vi "histogram_lifetimes.vi"(8 "error in (no error)":errorcluster, 11 "swabian_local_data 2":T1={"events"={"update_status"=refnum, "update_chart"=refnum, "update_xy"=refnum, "send_channel_data"=refnum}, "stop_q"=refnum, "tagger_reference"=refnum, "connect_button"=refnum, "counter_reference"=refnum, "tagger_stream_reference"=refnum, "log_reference"=refnum, "current_log_offset"=0, "tt20_buffer_q"=refnum, "stream_to_file_button"=refnum, "num_records"=0, "connected?"=FALSE, "plots"=refnum, "histogram_bin_edges"=[], "histogrammer"=refnum, "plot_lifetimes"=refnum, "xy_graph"=refnum, "Reference\nChannel"=enum."ch0", "trigger_channels"=[], "filter_channels"=[], "active_channels"=[], "acq_mode"=0, "Reference\nChannel"=enum."ch0", "acq_time"=0, "sync_period_ps"=0, "raw_stream_path"=path "", "Leftovers"={"missing_sync_data"=[], "missing_events"=0}, "first_batch"=0, "first_sync_stamp"=0, "lifetime_settings"={"Plot Lifetimes"=FALSE, "start_time"=0.0, "stop_time"=0.0, "n_bins"=0, "Oscilloscope"=TRUE}, "Histogram_bins"=[], "last_processed_data"=[], "histogram_data"=[]}) -> (0 "error out":errorcluster, 3 "swabian_local_data 3":T1={"events"={"update_status"=refnum, "update_chart"=refnum, "update_xy"=refnum, "send_channel_data"=refnum}, "stop_q"=refnum, "tagger_reference"=refnum, "connect_button"=refnum, "counter_reference"=refnum, "tagger_stream_reference"=refnum, "log_reference"=refnum, "current_log_offset"=0, "tt20_buffer_q"=refnum, "stream_to_file_button"=refnum, "num_records"=0, "connected?"=FALSE, "plots"=refnum, "histogram_bin_edges"=[], "histogrammer"=refnum, "plot_lifetimes"=refnum, "xy_graph"=refnum, "Reference\nChannel"=enum."ch0", "trigger_channels"=[], "filter_channels"=[], "active_channels"=[], "acq_mode"=0, "Reference\nChannel"=enum."ch0", "acq_time"=0, "sync_period_ps"=0, "raw_stream_path"=path "", "Leftovers"={"missing_sync_data"=[], "missing_events"=0}, "first_batch"=0, "first_sync_stamp"=0, "lifetime_settings"={"Plot Lifetimes"=FALSE, "start_time"=0.0, "stop_time"=0.0, "n_bins"=0, "Oscilloscope"=TRUE}, "Histogram_bins"=[], "last_processed_data"=[], "histogram_data"=[]})   [LabVIEW 2018]
uses:
  swabian_local_data_tdef.ctl
  swabian_events_tdef.ctl
  update_chart_tdef.ctl
  channel_data_tdef.ctl
  C:/Users/SWIR TCSPC/Documents/swabian_LV/lib/TTCSharp32.dll
  lib/TTCSharp32.dll
  swabian_buffer_tdef.ctl
  reference_checkbox_tdef.ctl
  lifetime_settings.ctl
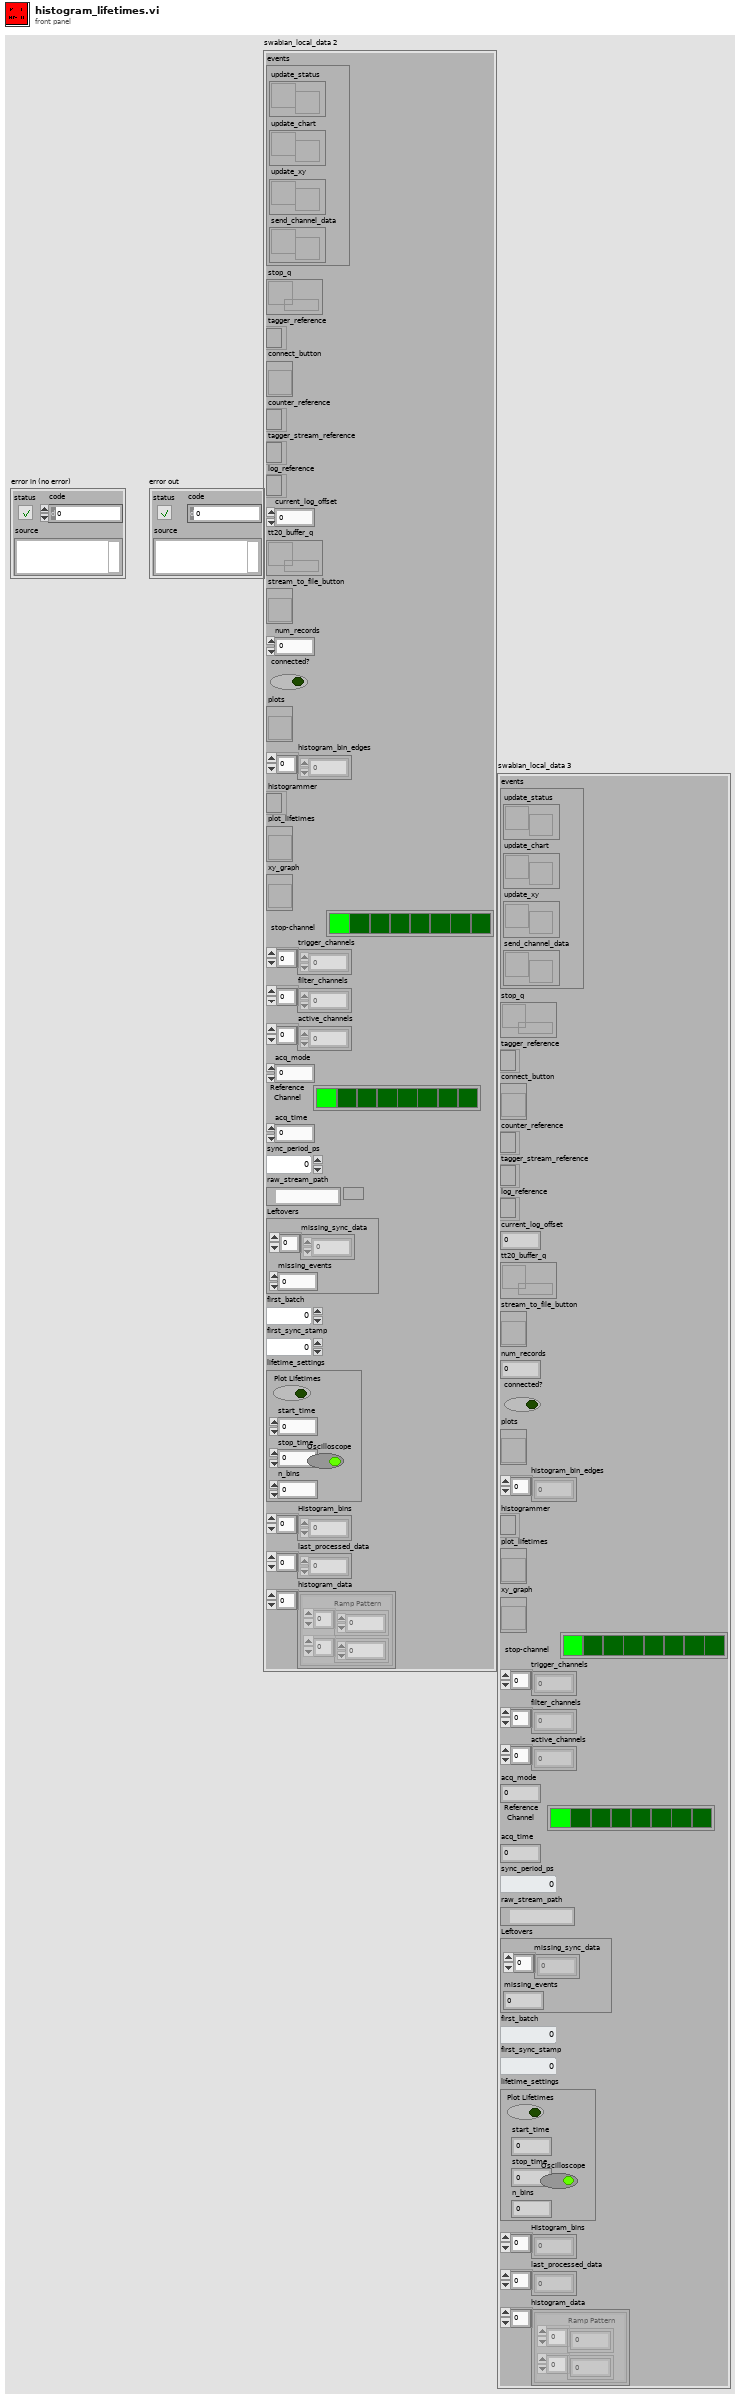
[diagram p1: front panel]
types:
  T1 = typedef "swabian_local_data_tdef.ctl" = cluster{"events":T2, "stop_q":refnum<queue>, "tagger_reference":refnum<k24>, "connect_button":refnum<vi>, "counter_reference":refnum<k24>, "tagger_stream_reference":refnum<k24>, "log_reference":refnum<file>, "current_log_offset":i64, "tt20_buffer_q":refnum<queue>, "stream_to_file_button":refnum<vi>, "num_records":u64, "connected?":bool, "plots":refnum<vi>, "histogram_bin_edges":i64[], "histogrammer":refnum<k24>, "plot_lifetimes":refnum<vi>, "xy_graph":refnum<vi>, "Reference\nChannel":T3, "trigger_channels":i32[], "filter_channels":i32[], "active_channels":i32[], "acq_mode":i32, "Reference\nChannel":T3, "acq_time":i64, "sync_period_ps":i64, "raw_stream_path":path, "Leftovers":cluster{"missing_sync_data":i64[], "missing_events":i32}, "first_batch":i32, "first_sync_stamp":i64, "lifetime_settings":T4, "Histogram_bins":dbl[], "last_processed_data":i64[], "histogram_data":cluster{"Ramp Pattern":dbl[], dbl[]}[]}
  T2 = typedef "swabian_events_tdef.ctl" = cluster{"update_status":refnum<user-event>, "update_chart":refnum<user-event>, "update_xy":refnum<user-event>, "send_channel_data":refnum<user-event>}
  T3 = typedef "reference_checkbox_tdef.ctl" = enum32{"No Selection", "ch0", "ch1", "ch2", "ch3", "ch4", "ch5", "ch6", "ch7"}
  T4 = typedef "lifetime_settings.ctl" = cluster{"Plot Lifetimes":bool, "start_time":dbl, "stop_time":dbl, "n_bins":i32, "Oscilloscope":bool}
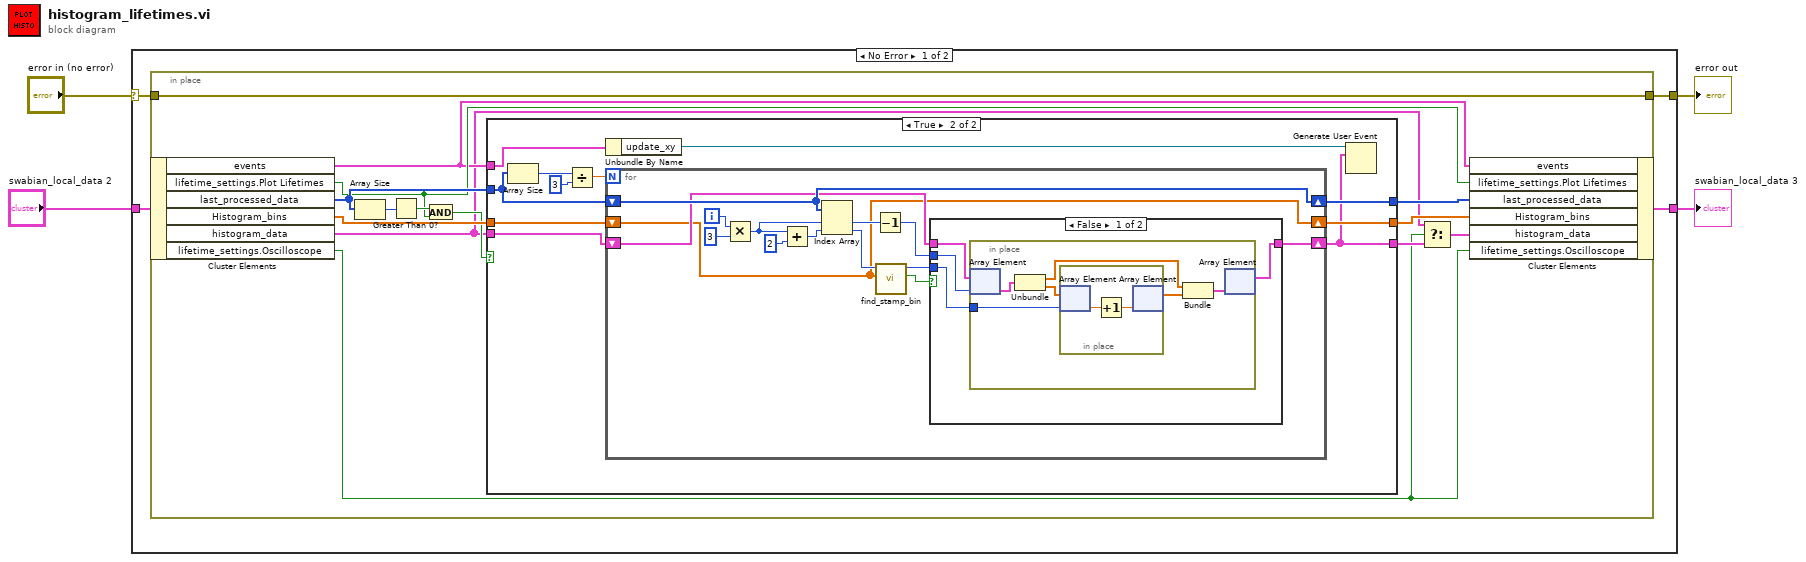
[diagram p0: block diagram]
diagram:
  n1 = case shown="No Error" "error in (no error)" {
    selector: "error in (no error)" -> [w7 w65]
    tunnel: "swabian_local_data 2" -> [w8 w64]
    tunnel: [w6 w65] -> w2
    tunnel: [w5 w64] -> w1
    frame No Error {
      n2 = in-place {
        in-place-border: w7 -> [w22]
        in-place-border: [w22] -> w6
        n3 = in-place-cluster #1(w8) -> ("events"=w13:T2, "lifetime_settings.Plot Lifetimes"=w15:bool, "last_processed_data"=w18:i64[], "Histogram_bins"=w21:dbl[], "histogram_data"=w10:cluster{"Ramp Pattern":dbl[], dbl[]}[], "lifetime_settings.Oscilloscope"=w9:bool)
        n4 = Array Size(array=w18) -> (size(s)=w17:i32)
        n5 = Greater Than 0?(x=w17) -> (x > 0?=w16:bool)
        n6 = And(x=w16, y=w15) -> (x .and. y?=w14:bool)
        n7 = case shown="True" w14 {
          tunnel: w13 -> [_ w36]
          tunnel: w18 -> [w25 w31]
          tunnel: w21 -> [w24 w30]
          tunnel: [w24 w29] -> w20
          tunnel: [w25 w28] -> w19
          tunnel: w10 -> [w23 w27]
          tunnel: [w23 w26] -> w12
          frame False {
          }
          frame True {
            n8 = Array Size(array=w31) -> (size(s)=w34:i32)
            n9 = Divide(x=w34, y=3) -> (x/y=w32:dbl)
            n10 = Unbundle By Name(w36) -> ("update_xy"=w35:refnum<user-event>)
            n11 = for {
              N: w32 -> [_]
              shift-right: [w50] -> w28
              shift-left: w31 -> [w50]
              shift-right: [w38] -> w29
              shift-left: w30 -> [w38]
              shift-right: [w39] -> w26
              shift-left: w27 -> [w41]
              i -> [w49]
              n12 = Multiply(x=w49, y=3) -> (x*y=w47:i32)
              n13 = Add(x=w47, y=2) -> (x+y=w45:i32)
              n14 = Index Array(array=w50, index #1=w47, index #2=w45) -> (element #1=w43:i64, element #2=w44:i64)
              n15 = Decrement(x=w43) -> (x-1=w42:i64)
              n16 = call "find_stamp_bin.vi"("Histogram_bins"=w38, "stamp"=w44) -> ("out_of_bounds"=w37:bool, "bin"=w40:i32)  [unwired: 8 in]
              n17 = case shown="False" w37 {
                tunnel: w42 -> [w54 _]
                tunnel: w41 -> [w53 w63]
                tunnel: w40 -> [w52 _]
                tunnel: [w51 w63] -> w39
                frame False {
                  n18 = in-place {
                    in-place-border: w52 -> [w57]
                    n19 = in-place-array #2(w53, w54) -> (w60:cluster{"Ramp Pattern":dbl[], dbl[]})
                    n20 = Unbundle(w60) -> ("Ramp Pattern"=w59:dbl[], w58:dbl[])
                    n21 = in-place {
                      n22 = in-place-array #3(w58, w57) -> (w62:dbl)
                      n23 = Increment(x=w62) -> (x+1=w61:dbl)
                      n24 = in-place-array #3(w61) -> (w56:dbl[])  [unwired: 1 out]
                    }
                    n25 = Bundle("Ramp Pattern"=w59, w56) -> (w55:cluster{"Ramp Pattern":dbl[], dbl[]})  [unwired: 1 in]
                    n26 = in-place-array #2(w55) -> (w51:cluster{"Ramp Pattern":dbl[], dbl[]}[])  [unwired: 1 out]
                  }
                }
                frame True {
                }
              }
            }
            n27 = Generate User Event(user event=w35, event data cluster=w26) -> ()  [unwired: 2 in, 2 out]
          }
        }
        n28 = Select(t=w10, s=w9, f=w12) -> (s? t:f=w11:cluster{"Ramp Pattern":dbl[], dbl[]}[])
        n29 = in-place-cluster #1("events"=w13, "lifetime_settings.Plot Lifetimes"=w15, "last_processed_data"=w19, "Histogram_bins"=w20, "histogram_data"=w11, "lifetime_settings.Oscilloscope"=w9) -> (w5:T1)
      }
    }
    frame Error {
    }
  }
  "error out" <- w2
  "swabian_local_data 3" <- w1
